vi "Collision_code_Testing.vi"() -> ()   [LabVIEW 2022 SP3]
uses:
  EnFlo specific/Collision Mode.ctl
  EnFlo specific/Collision Detection global.vi
panel:
  in  "Traverse Active Parts":cluster{"X":bool, "XY":bool, "XYZ":bool}
  out "Traverse collision part":cluster{"X":bool, "XY":bool, "XYZ":bool}
  out "Collision":bool
  out "Minimum separation":sgl
  out "Minimum separation vector (from trav.)":sgl[](array[numeric])
  in  "3D graphics output":bool=TRUE
  in  "Get minimum separation within look-out sphere":bool=TRUE
  in  "Collision mode":T1=enum."Traverse - All"
  in  "Traverse position (absolute, mm)":sgl[](array[numeric])=[0.0, 0.0, 150.0]
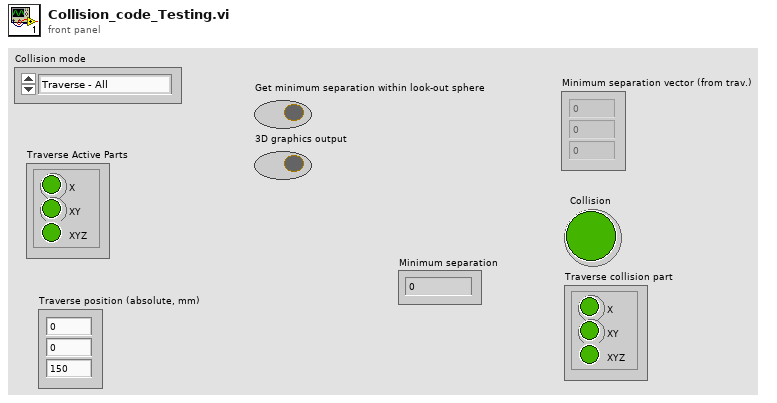
[diagram p1: front panel]
types:
  T1 = typedef "Collision Mode.ctl" = enum16{"Traverse - Tunnel", "Traverse - Model", "Traverse - Fixed objects", "Traverse - Traverse", "Traverse - All"}
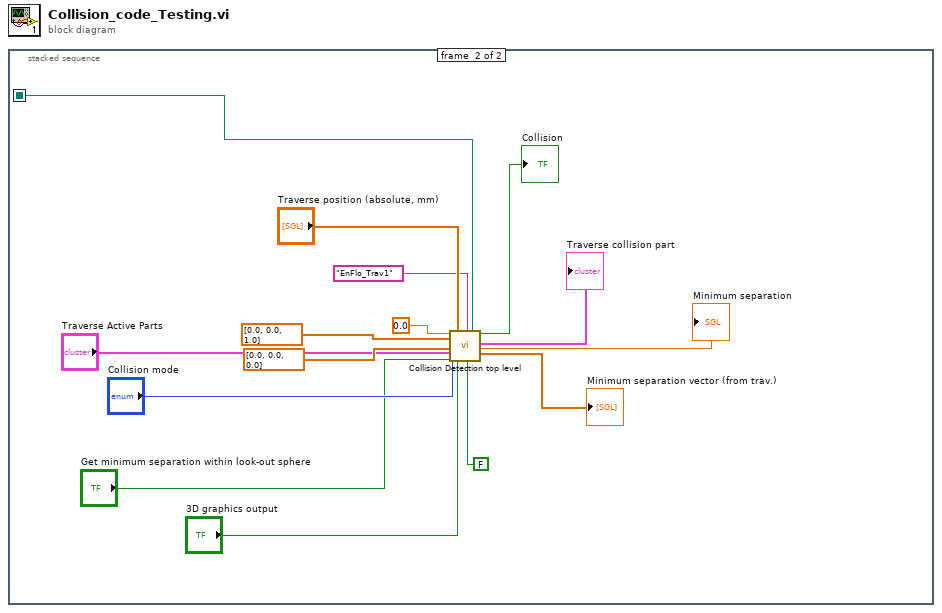
[diagram p0: block diagram]
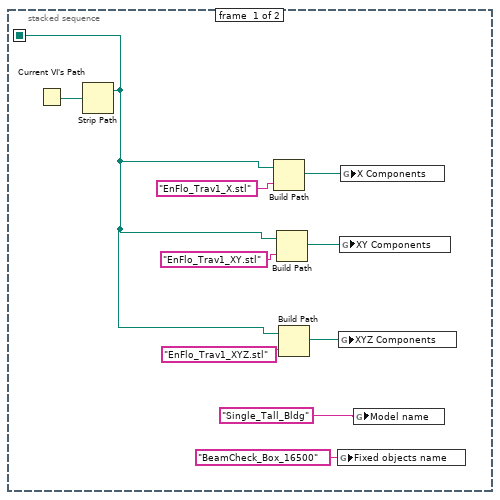
[diagram p2: hidden frame]
diagram:
  n1 = stacked-sequence {
    seq-local: [w2 _] -> [_ w16]
    frame #0 {
      n2 = Current VI's Path() -> (path=w10:path)
      n3 = Strip Path(path=w10) -> (stripped path=w2:path)  [unwired: 1 out]
      n4 = Build Path(base path=w2, name or relative path="EnFlo_Trav1_X.stl") -> (appended path=w8:path)
      n5 = Build Path(base path=w2, name or relative path="EnFlo_Trav1_XY.stl") -> (appended path=w7:path)
      n6 = Build Path(base path=w2, name or relative path="EnFlo_Trav1_XYZ.stl") -> (appended path=w4:path)
      n7 = global write "Collision Detection global.vi" "Fixed objects name"("BeamCheck_Box_16500" ("Fixed objects name")) -> ()
      n8 = global write "Collision Detection global.vi" "XYZ Components"(w4) -> ()
      n9 = global write "Collision Detection global.vi" "XY Components"(w7) -> ()
      n10 = global write "Collision Detection global.vi" "X Components"(w8) -> ()
      n11 = global write "Collision Detection global.vi" "Model name"("Single_Tall_Bldg") -> ()
    }
    frame #1 {
      n12 = call "Collision Detection top level.vi"("Model rotation (degrees)"=sgl 0.0, "Model rotation axis (unit vector)"=sgl[] [0.0, 0.0, 1.0], "Traverse Active Parts"="Traverse Active Parts", "Model rotation axis coordinates (absolute, mm)"=sgl[] [0.0, 0.0, 0.0], "Collision mode"="Collision mode", "Get minimum separation within look-out sphere"="Get minimum separation within look-out sphere", "Traverse position (absolute, mm)"="Traverse position (absolute, mm)", "3D graphics output"="3D graphics output", "Traverse name"="EnFlo_Trav1", "Extrusion mode"=FALSE, "Rig geometry directory path"=w16) -> ("Collision"=→"Collision":bool, "Traverse collision part"=→"Traverse collision part":cluster{"X":bool, "XY":bool, "XYZ":bool}, "Minimum separation"=→"Minimum separation":sgl, "Minimum separation vector (from trav.)"=→"Minimum separation vector (from trav.)":sgl[])  [unwired: 3 in, 2 out]
    }
  }
